vi "Read All Elements.vi"(8 "error in (no error)":errorcluster, 11 "Look Up Table in":refnum<class "Look Up Table.lvclass">) -> (0 "error out":errorcluster, 1 "All Elements":variant[](array[variant]), 2 "Names":string[](array[string]), 3 "Look Up Table out":refnum<class "Look Up Table.lvclass">)   [LabVIEW 2016, in "Stream Look Up Table.lvlib" / "Look Up Table.lvclass"]
doc: "--\nCopyright © 2017 Composed SystemsI All rights reserved.\n\nAuthor: Jon McBee <jon.mcbee@composed.io>\n\nThis library is provided \"AS IS\" ,WITHOUT WARRANTIES OR\nCONDITIONS OF ANY KIND, either express or implied.\n\nComposed Systems -- composed.io\n\nStream 0.0.1.1\nJon McBee - Composed Systems\nCopyright (c) 2017, Composed Systems"
uses:
  <userlib>/Composed Systems/Stream/Look Up Table/Look Up Table/Look Up Table.lvclass
  <userlib>/Composed Systems/Stream/Look Up Table/Look Up Table/Look Up Table.lvclass/Look Up Table.ctl
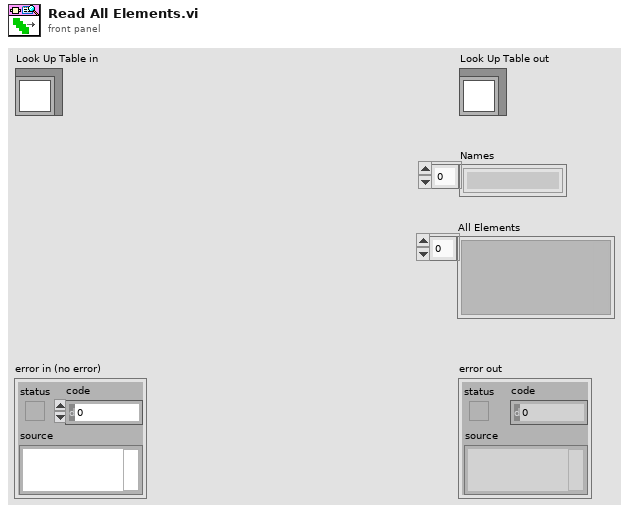
[diagram p1: front panel]
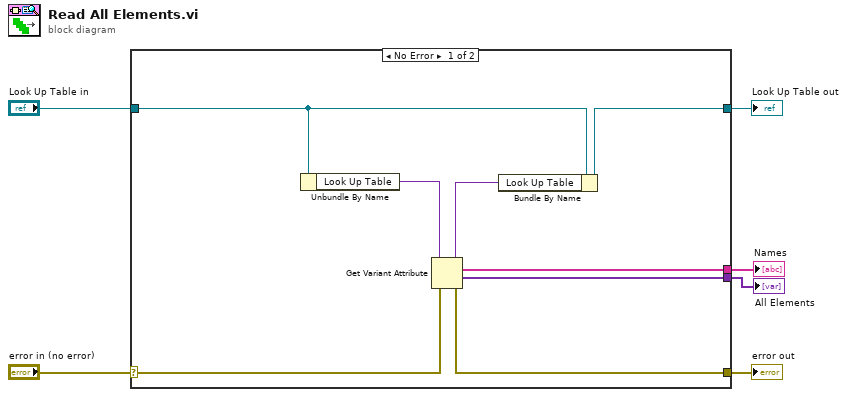
[diagram p0: block diagram]
diagram:
  n1 = case shown="No Error" "error in (no error)" {
    selector: "error in (no error)" -> [w10 w16]
    tunnel: [w9 w16] -> w5
    tunnel: [w11 w15] -> w3
    tunnel: "Look Up Table in" -> [w12 w15]
    tunnel: [w8 _] -> w2
    tunnel: [w7 _] -> w1
    frame No Error {
      n2 = Unbundle By Name(w12) -> ("Look Up Table"=w14:variant)
      n3 = Get Variant Attribute(Variant=w14, error in=w10) -> (duplicate Variant=w13:variant, names=w8:string[], values=w7:variant[], error out=w9:errorcluster)  [unwired: 2 in]
      n4 = Bundle By Name(cluster=w12, "Look Up Table"=w13) -> (w11:refnum<class "Look Up Table.lvclass">)
    }
    frame Error {
    }
  }
  "error out" <- w5
  "Look Up Table out" <- w3
  "Names" <- w2
  "All Elements" <- w1
